vi "Solver_010.vi"(10 "Word List":string[](array[string])=["YELLOW", "ORANGE", "PURPLE", "BLUE", "GREEN", "RED"], 11 "Word Search Grid":string[][](array[string])=[["R", "B", "L", "U", "E", "W"], ["E", "G", "N", "A", "R", "O"], ["D", "B", "C", "E", "W", "L"], ["L", "L", "D", "K", "V", "L"], ["P", "U", "R", "P", "L", "E"], ["N", "E", "E", "R", "G", "Y"]]) -> (3 "Solutions":T1={"BLUE"=[{"Row"=0, "Column"=1}, {"Row"=0, "Column"=2}, {"Row"=0, "Column"=3}, {"Row"=0, "Column"=4}], "GREEN"=[{"Row"=5, "Column"=4}, {"Row"=5, "Column"=3}, {"Row"=5, "Column"=2}, {"Row"=5, "Column"=1}, {"Row"=5, "Column"=0}], "ORANGE"=[{"Row"=1, "Column"=5}, {"Row"=1, "Column"=4}, {"Row"=1, "Column"=3}, {"Row"=1, "Column"=2}, {"Row"=1, "Column"=1}, {"Row"=1, "Column"=0}], "PURPLE"=[{"Row"=4, "Column"=0}, {"Row"=4, "Column"=1}, {"Row"=4, "Column"=2}, {"Row"=4, "Column"=3}, {"Row"=4, "Column"=4}, {"Row"=4, "Column"=5}], "RED"=[{"Row"=0, "Column"=0}, {"Row"=1, "Column"=0}, {"Row"=2, "Column"=0}], "YELLOW"=[{"Row"=5, "Column"=5}, {"Row"=4, "Column"=5}, {"Row"=3, "Column"=5}, {"Row"=2, "Column"=5}, {"Row"=1, "Column"=5}, {"Row"=0, "Column"=5}]})   [LabVIEW 2022 SP3]
uses:
  Solutions--map.ctl
  Letter Index--cluster.ctl
panel:
  out "index of element 2":i32
  out "index of element":i32
  out "Array":string[][](array[string])
  out "output array 2":string[](array[string])
  out "output array":string[](array[string])
  # "Do not change the connector pane of this VI."
  # "Observe the default values stored in this VI to understand how each word is represented in the Solutions map.\n\nSee the block diagram for a simple implementation of a solution. Note that this approach is not very efficient, and you will want to come up with a faster way to find the words in the grid."
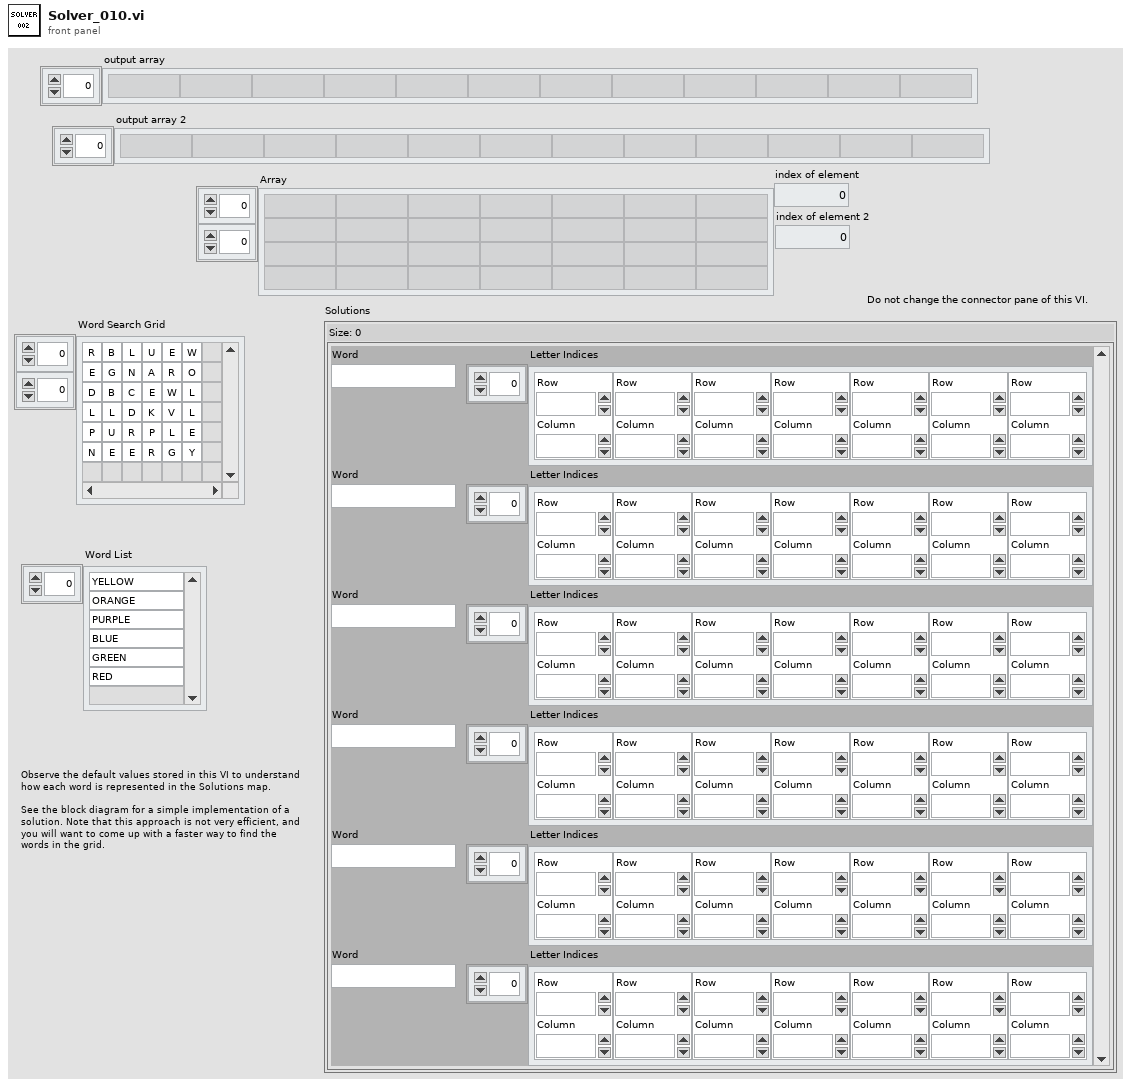
[diagram p1: front panel]
types:
  T1 = typedef "Solutions--map.ctl" = map{string, T2[]}
  T2 = typedef "Letter Index--cluster.ctl" = cluster{"Row":i32, "Column":i32}
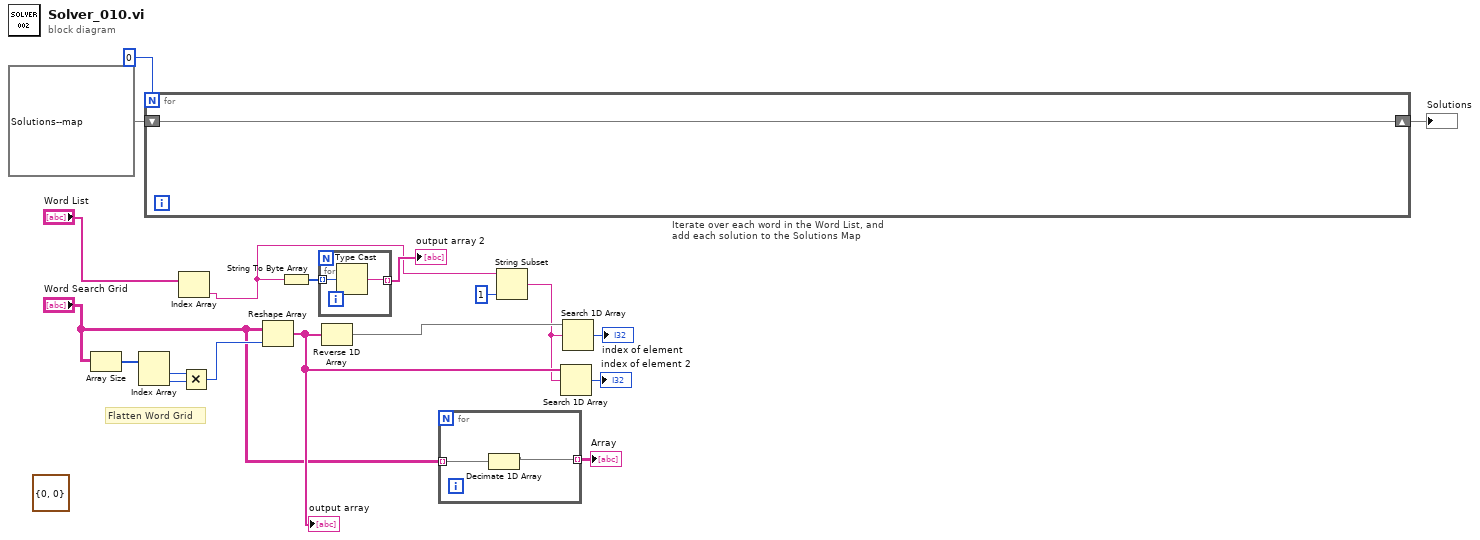
[diagram p0: block diagram]
diagram:
  (unwired) T2 {"Row"=0, "Column"=0} ("Letter Index")
  # "Flatten Word Grid"
  n1 = Array Size(array="Word Search Grid") -> (size(s)=w15:i32[])
  n2 = Index Array(array=w15) -> (element #1=w14:i32, element #2=w13:i32)  [unwired: 2 in]
  n3 = for "Iterate over each word in the Word List, and add each solution to the Solutions Map" {
    N: 0 -> [_]
    shift-right: [w20] -> w19
    shift-left: T1 {} ("Solutions") -> [w20]
  }
  "Solutions" <- w19
  n4 = Index Array(array="Word List") -> (element=w7:string)  [unwired: 1 in]
  n5 = Multiply(x=w14, y=w13) -> (x*y=w12:i32)
  n6 = Reshape Array("Word Search Grid", w12) -> (w8:string[])
  "output array" <- w8
  n7 = String To Byte Array(string=w7) -> (unsigned byte array=w11:u8[])
  n8 = for {
    tunnel: w11 -> [w21] mode=indexing
    tunnel: [w22] -> w9 mode=indexing
    n9 = Type Cast(x=w21) -> (*(type *) &x=w22:string)  [unwired: 1 in]
  }
  "output array 2" <- w9
  n10 = Reverse 1D Array(array=w8) -> (reversed array=w10:string[])
  n11 = for {
    tunnel: "Word Search Grid" -> [w24] mode=indexing
    tunnel: [w23] -> w4 mode=indexing
    n12 = Decimate 1D Array(w24) -> (w23:string[])  [unwired: 1 out]
  }
  "Array" <- w4
  n13 = String Subset(string=w7, length (rest)=1 ("length (rest)")) -> (substring=w3:string)  [unwired: 1 in]
  n14 = Search 1D Array(1D array=w8, element=w3) -> (index of element=→"index of element 2":i32)  [unwired: 1 in]
  n15 = Search 1D Array(1D array=w10, element=w3) -> (index of element=→"index of element":i32)  [unwired: 1 in]
